vi "testingCode.vi"() -> ()   [LabVIEW 2020]
uses:
  C:/Users/DESKTOP-TLO0G68A/Desktop/LabVIEW/instrumentationLV/ThorLabs.MotionControl.KCube.DCServoCLI.dll
  ThorLabs.MotionControl.KCube.DCServoCLI.dll
  C:/Users/DESKTOP-TLO0G68A/Desktop/LabVIEW/instrumentationLV/Thorlabs.MotionControl.GenericMotorCLI.dll
  Thorlabs.MotionControl.GenericMotorCLI.dll
  C:/Users/DESKTOP-TLO0G68A/Desktop/LabVIEW/instrumentationLV/Thorlabs.MotionControl.Controls.dll
  Thorlabs.MotionControl.Controls.dll
panel:
  in  "stepSize":dbl
  in  "SerialNumber":string="27502753"
  in  "KCubeDCServoControl":refnum<k24>(container)
  in  "x steps":i32
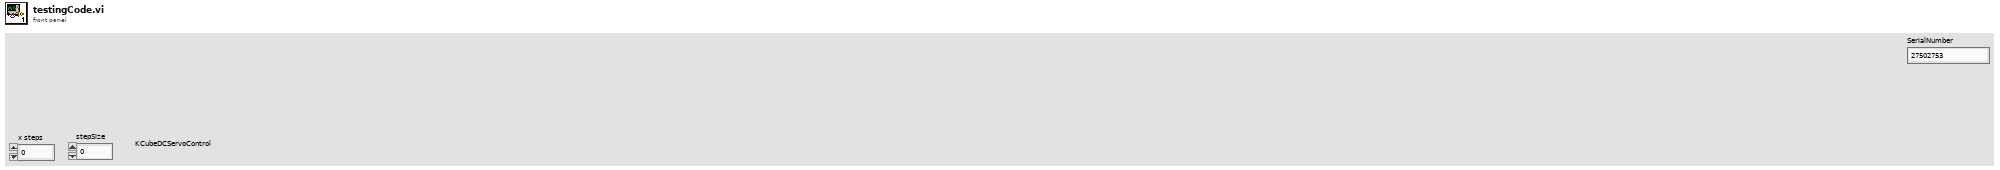
[diagram p1: front panel]
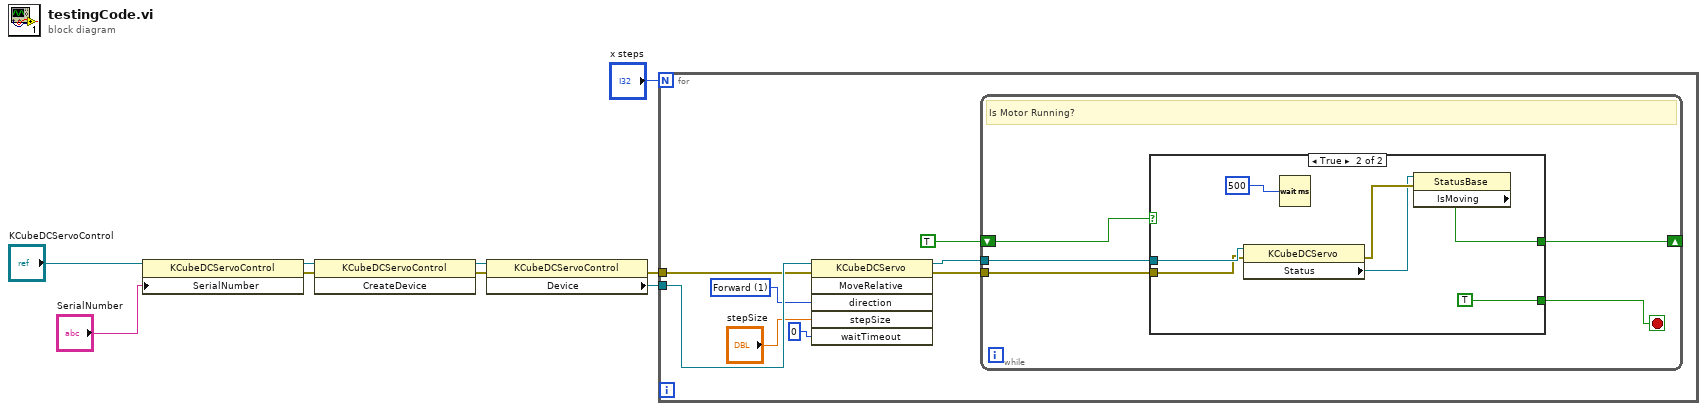
[diagram p0: block diagram]
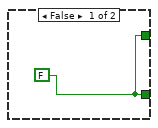
[diagram p2: hidden frame]
diagram:
  n1 = property class="KCubeDCServoControl"(reference="KCubeDCServoControl", "SerialNumber"="SerialNumber") -> (reference out=w7:refnum<k24>, error out=w5:errorcluster)  [unwired: 1 in]
  n2 = invoke class="KCubeDCServoControl" method="CreateDevice"(reference=w7, error in=w5) -> (reference out=w6:refnum<k24>, error out=w4:errorcluster)  [unwired: 1 in, 1 out]
  n3 = property class="KCubeDCServoControl"(reference=w6, error in=w4) -> (error out=w1:errorcluster, "Device"=w2:refnum<k24>)  [unwired: 1 out]
  n4 = for {
    N: "x steps" -> [_]
    tunnel: w2 -> [w16]
    tunnel: w1 -> [w15]
    w13 = 1 items=["Forward"=1, "Backward"=2] ("direction")
    n5 = invoke class="KCubeDCServo" method="MoveRelative"(reference=w16, error in=w15, "direction"=w13, "stepSize"="stepSize", "waitTimeout"=0) -> (reference out=w11:refnum<k24>, error out=w10:errorcluster)  [unwired: 1 in, 4 out]
    n6 = while {
      shift-right: [w21] -> _
      shift-left: TRUE -> [w22]
      tunnel: w11 -> [w20]
      tunnel: w10 -> [w19]
      stop <- w18 stop-if-true
      # "Is Motor Running?"
      n7 = case shown="True" w22 {
        tunnel: [w23 w30] -> w21
        tunnel: w20 -> [_ w27]
        tunnel: w19 -> [_ w26]
        tunnel: [w23 TRUE] -> w18
        frame False {
          w23 = FALSE
        }
        frame True {
          n8 = property class="KCubeDCServo"(reference=w27, error in=w26) -> (error out=w29:errorcluster, "Status"=w28:refnum<k24>)  [unwired: 1 out]
          n9 = Wait (ms)(milliseconds to wait=u32 500) -> ()  [unwired: 1 out]
          n10 = property class="StatusBase"(reference=w28, error in=w29) -> ("IsMoving"=w30:bool)  [unwired: 2 out]
        }
      }
    }
  }
